vi "Manual Motor Controller.vi"(4 "Curving\nFactor":dbl(slide)=0.5 scale=-1.0..1.0, 6 "Speed":dbl(slide) scale=0.0..1.0, 8 "Backward":bool, 9 "Right":bool, 10 "Left":bool, 11 "Forward":bool) -> (0 "Duty Cycle B2":dbl, 1 "Duty Cycle B1":dbl, 2 "Duty Cycle A2":dbl, 3 "Duty Cycle A1":dbl)   [LabVIEW 2019]
doc: "The motor controlling programmation for the Manual Drive.\nInputs Forward, Left, Right, Backward are booleans to indicate in which direction you would like to drive.\nInput Speed is to limit the speed at which the motors will turn.\nInput Curving Factor limits the speed of the slower motor during a curve (forward + left or right)."
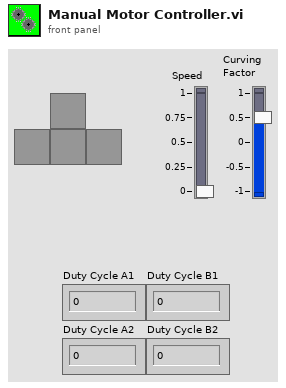
[diagram p1: front panel]
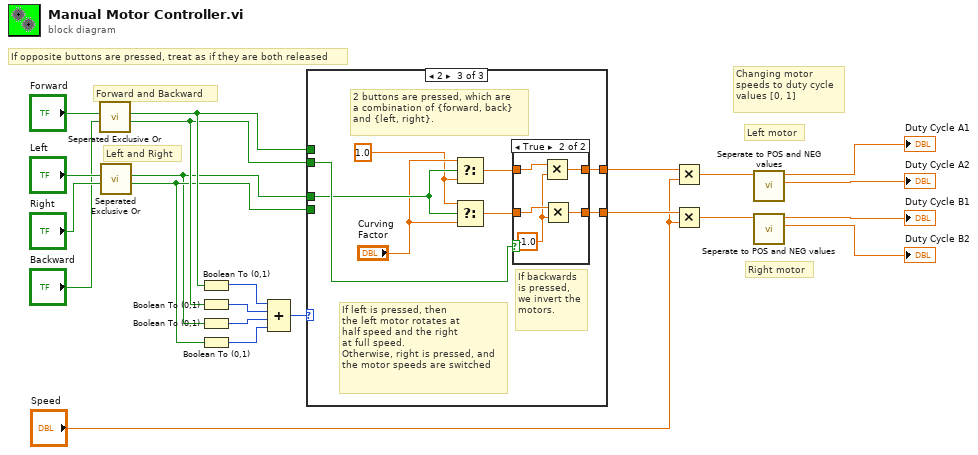
[diagram p0: block diagram]
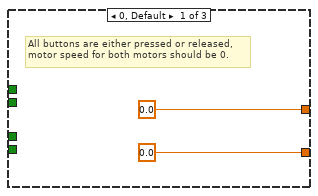
[diagram p2: hidden frame]
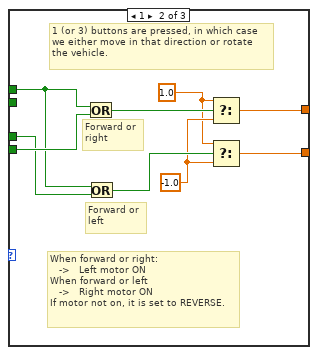
[diagram p3: hidden frame]
diagram:
  # "If opposite buttons are pressed, treat as if they are both released"
  # "Changing motor\nspeeds to duty cycle\nvalues [0, 1]"
  # "Right motor"
  # "Left motor"
  # "Left and Right"
  # "Forward and Backward"
  n1 = call "Seperated Exclusive Or.vi"("q"="Backward", "p"="Forward") -> ("only q"=w12:bool, "only p"=w13:bool)  [unwired: 8 in]
  n2 = call "Seperated Exclusive Or.vi"("q"="Right", "p"="Left") -> ("only q"=w11:bool, "only p"=w10:bool)  [unwired: 8 in]
  n3 = Boolean To (0,1)(Boolean=w13) -> (0, 1=w18:i16)
  n4 = Boolean To (0,1)(Boolean=w12) -> (0, 1=w17:i16)
  n5 = Boolean To (0,1)(Boolean=w10) -> (0, 1=w16:i16)
  n6 = Boolean To (0,1)(Boolean=w11) -> (0, 1=w15:i16)
  n7 = Compound Arithmetic op=ADD(w18, w17, w16, w15) -> (w14:i16)
  n8 = case shown="2" w14 {
    tunnel: [0.0 w32 w37] -> w8
    tunnel: [0.0 w33 w39] -> w9
    tunnel: w13 -> [_ w26 _]
    tunnel: w12 -> [_ _ w41]
    tunnel: w11 -> [_ w29 _]
    tunnel: w10 -> [_ w25 w36]
    frame 0, Default {
      # "All buttons are either pressed or released, \nmotor speed for both motors should be 0."
    }
    frame 1 {
      w28 = -1.0
      w27 = 1.0
      # "When forward or right:\n   ->   Left motor ON\nWhen forward or left\n   ->   Right motor ON\nIf motor not on, it is set to REVERSE."
      # "Forward or\nleft"
      # "Forward or\nright"
      # "1 (or 3) buttons are pressed, in which case\nwe either move in that direction or rotate\nthe vehicle."
      n9 = Or(x=w26, y=w29) -> (x .or. y?=w31:bool)
      n10 = Or(x=w26, y=w25) -> (x .or. y?=w30:bool)
      n11 = Select(t=w27, s=w31, f=w28) -> (s? t:f=w33:dbl)
      n12 = Select(t=w27, s=w30, f=w28) -> (s? t:f=w32:dbl)
    }
    frame 2 {
      w34 = 1.0
      # "If left is pressed, then\nthe left motor rotates at\nhalf speed and the right\nat full speed.\nOtherwise, right is pressed, and\nthe motor speeds are switched"
      # "If backwards\nis pressed,\nwe invert the\nmotors."
      # "2 buttons are pressed, which are\na combination of {forward, back}\nand {left, right}."
      n13 = Select(t="Curving\nFactor", s=w36, f=w34) -> (s? t:f=w40:dbl)
      n14 = Select(t=w34, s=w36, f="Curving\nFactor") -> (s? t:f=w38:dbl)
      n15 = case shown="True" w41 {
        tunnel: w40 -> [w43 w48]
        tunnel: [w43 w47] -> w39
        tunnel: w38 -> [w42 w46]
        tunnel: [w42 w44] -> w37
        frame False {
        }
        frame True {
          w45 = -1.0
          n16 = Multiply(x=w48, y=w45) -> (x*y=w47:dbl)
          n17 = Multiply(x=w46, y=w45) -> (x*y=w44:dbl)
        }
      }
    }
  }
  n18 = Multiply(x=w9, y="Speed") -> (x*y=w6:dbl)
  n19 = Multiply(x=w8, y="Speed") -> (x*y=w5:dbl)
  n20 = call "Seperate to POS and NEG values.vi"("Motorspeed"=w6) -> ("Duty Cycle 2"=→"Duty Cycle A2":dbl, "Duty Cycle 1"=→"Duty Cycle A1":dbl)  [unwired: 9 in]
  n21 = call "Seperate to POS and NEG values.vi"("Motorspeed"=w5) -> ("Duty Cycle 2"=→"Duty Cycle B2":dbl, "Duty Cycle 1"=→"Duty Cycle B1":dbl)  [unwired: 9 in]
